vi "CH1_Comm_Stream.vi"   [LabVIEW 2018]
uses:
  RxTx/RxTx.lvclass
  Stream/Stream.lvclass
  Stream/Stream.lvclass/Stream.ctl
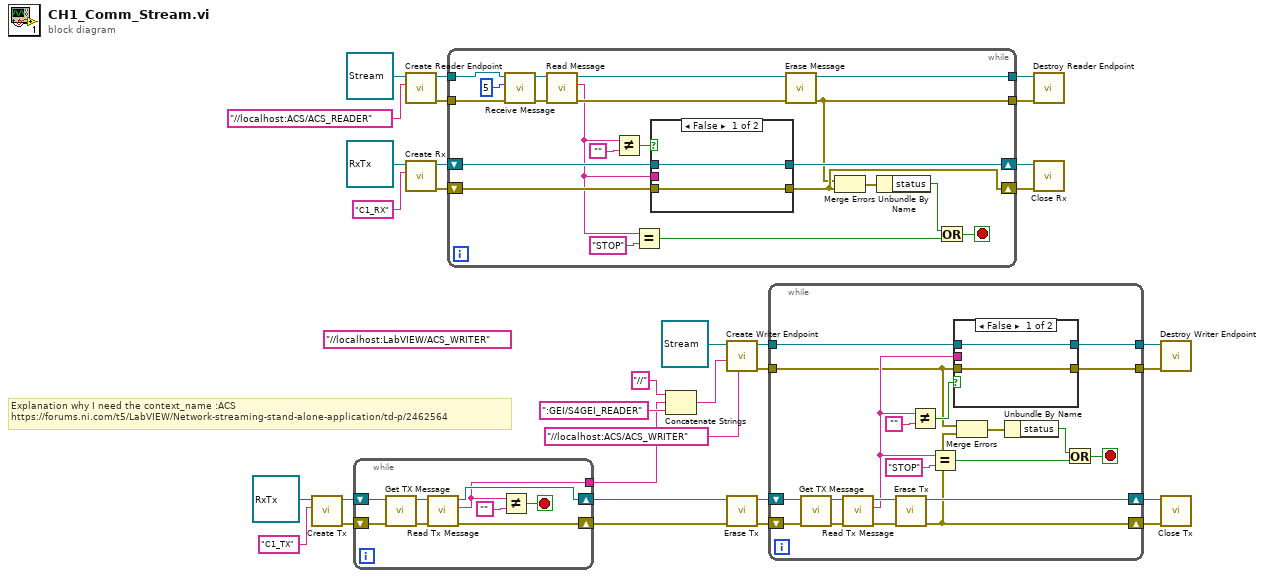
[diagram p0: block diagram]
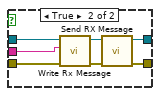
[diagram p2: hidden frame]
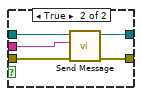
[diagram p3: hidden frame]
diagram:
  (unwired) "//localhost:LabVIEW/ACS_WRITER" ("reader name")
  # "Explanation why I need the context_name :ACS\nhttps://forums.ni.com/t5/LabVIEW/Network-streaming-stand-alone-application/td-p/2462564"
  n1 = call "Create Tx.vi"("Writer Name"="C1_TX", "RxTx in"=refnum<class "RxTx.lvclass"> refnum ("RxTx.lvclass")) -> ("error out"=w3:errorcluster, "RxTx out"=w2:refnum<class "RxTx.lvclass">)  [unwired: 8 in]
  n2 = while {
    shift-right: [w39] -> w4
    shift-left: w2 -> [w41]
    shift-right: [w38] -> w5
    shift-left: w3 -> [w36]
    tunnel: [w33] -> w1
    stop <- w34 stop-if-true
    n3 = call "Get TX Message.vi"("error in (no error)"=w36, "RxTx in"=w41) -> ("error out"=w37:errorcluster, "RxTx out"=w40:refnum<class "RxTx.lvclass">)  [unwired: 8 in]
    n4 = call "Read Tx Message.vi"("error in (no error)"=w37, "RxTx in"=w40) -> ("error out"=w38:errorcluster, "Tx Message"=w33:string, "RxTx out"=w39:refnum<class "RxTx.lvclass">)  [unwired: 7 in]
    n5 = Not Equal?(x=w33, y="") -> (x != y?=w34:bool)
  }
  n6 = call "Create Reader Endpoint.vi"("reader name"="//localhost:ACS/ACS_READER", "Stream in"=refnum<class "Stream.lvclass"> refnum) -> ("error out"=w25:errorcluster, "Stream out"=w26:refnum<class "Stream.lvclass">)  [unwired: 8 in]
  n7 = call "Create Rx.vi"("Reader Name"="C1_RX", "RxTx in"=refnum<class "RxTx.lvclass"> refnum ("RxTx.lvclass")) -> ("error out"=w11:errorcluster, "RxTx out"=w12:refnum<class "RxTx.lvclass">)  [unwired: 8 in]
  n8 = while {
    shift-right: [w60] -> w29
    shift-left: w12 -> [w62]
    shift-right: [w46] -> w30
    shift-left: w11 -> [w61]
    tunnel: w26 -> [w59]
    tunnel: w25 -> [w58]
    tunnel: [w52] -> w24
    tunnel: [w45] -> w23
    stop <- w42 stop-if-true
    n9 = call "Receive Message.vi"("error in (no error)"=w58, "timeout ms"=5, "Stream in"=w59) -> ("error out"=w55:errorcluster, "Stream out"=w56:refnum<class "Stream.lvclass">)  [unwired: 7 in]
    n10 = call "Read Message.vi"("error in (no error)"=w55, "Stream in"=w56) -> ("error out"=w53:errorcluster, "Message"=w48:string, "Stream out"=w54:refnum<class "Stream.lvclass">)  [unwired: 7 in]
    n11 = Not Equal?(x=w48, y="") -> (x != y?=w50:bool)
    n12 = Equal?(x=w48, y="STOP" ("reader name")) -> (x = y?=w47:bool)
    n13 = case shown="False" w50 {
      tunnel: w62 -> [w64 w71]
      tunnel: w61 -> [w63 w68]
      tunnel: [w63 w67] -> w46
      tunnel: [w64 w66] -> w60
      tunnel: w48 -> [_ w65]
      frame False {
      }
      frame True {
        n14 = call "Write Rx Message.vi"("error in (no error)"=w68, "Rx Message"=w65, "RxTx in"=w71) -> ("error out"=w69:errorcluster, "RxTx out"=w70:refnum<class "RxTx.lvclass">)  [unwired: 7 in]
        n15 = call "Send RX Message.vi"("error in (no error)"=w69, "RxTx in"=w70) -> ("error out"=w67:errorcluster, "RxTx out"=w66:refnum<class "RxTx.lvclass">)  [unwired: 8 in]
      }
    }
    n16 = call "Erase Message.vi"("error in (no error)"=w53, "Stream in"=w54) -> ("error out"=w45:errorcluster, "Stream out"=w52:refnum<class "Stream.lvclass">)  [unwired: 8 in]
    n17 = Merge Errors(w45, w46) -> (w44:errorcluster)
    n18 = Unbundle By Name(w44) -> ("status"=w43:bool)
    n19 = Or(x=w43, y=w47) -> (x .or. y?=w42:bool)
  }
  n20 = Concatenate Strings("//" ("reader name"), w1, ":GEI/S4GEI_READER" ("reader name")) -> (w9:string)
  n21 = call "Create Writer Endpoint.vi"("writer name"="//localhost:ACS/ACS_WRITER" ("reader name"), "reader name"=w9, "Stream in"=refnum<class "Stream.lvclass"> refnum) -> ("error out"=w21:errorcluster, "Stream out"=w22:refnum<class "Stream.lvclass">)  [unwired: 7 in]
  n22 = call "Erase Tx.vi"("error in (no error)"=w5, "RxTx in"=w4) -> ("error out"=w6:errorcluster, "RxTx out"=w7:refnum<class "RxTx.lvclass">)  [unwired: 8 in]
  n23 = while {
    shift-right: [w85] -> w31
    shift-left: w7 -> [w91]
    shift-right: [w74] -> w32
    shift-left: w6 -> [w90]
    tunnel: w22 -> [w82]
    tunnel: w21 -> [w73]
    tunnel: [w81] -> w20
    tunnel: [w80] -> w19
    stop <- w75 stop-if-true
    n24 = call "Get TX Message.vi"("error in (no error)"=w90, "RxTx in"=w91) -> ("error out"=w88:errorcluster, "RxTx out"=w89:refnum<class "RxTx.lvclass">)  [unwired: 8 in]
    n25 = call "Read Tx Message.vi"("error in (no error)"=w88, "RxTx in"=w89) -> ("error out"=w87:errorcluster, "Tx Message"=w79:string, "RxTx out"=w86:refnum<class "RxTx.lvclass">)  [unwired: 7 in]
    n26 = call "Erase Tx.vi"("error in (no error)"=w87, "RxTx in"=w86) -> ("error out"=w74:errorcluster, "RxTx out"=w85:refnum<class "RxTx.lvclass">)  [unwired: 8 in]
    n27 = Not Equal?(x=w79, y="") -> (x != y?=w83:bool)
    n28 = Equal?(x=w79, y="STOP") -> (x = y?=w77:bool)
    n29 = case shown="False" w83 {
      tunnel: w79 -> [_ w98]
      tunnel: w82 -> [w93 w97]
      tunnel: w73 -> [w92 w96]
      tunnel: [w92 w95] -> w81
      tunnel: [w93 w94] -> w80
      frame False {
      }
      frame True {
        n30 = call "Send Message.vi"("error in (no error)"=w96, "Message"=w98, "Stream in"=w97) -> ("error out"=w95:errorcluster, "Stream out"=w94:refnum<class "Stream.lvclass">)  [unwired: 7 in]
      }
    }
    n31 = Merge Errors(w73, w74) -> (w72:errorcluster)
    n32 = Unbundle By Name(w72) -> ("status"=w76:bool)
    n33 = Or(x=w76, y=w77) -> (x .or. y?=w75:bool)
  }
  n34 = call "Destroy Reader Endpoint.vi"("error in (no error)"=w23, "Stream in"=w24) -> ()  [unwired: 8 in, 2 out]
  n35 = call "Close Rx.vi"("error in (no error)"=w30, "RxTx in"=w29) -> ()  [unwired: 8 in, 2 out]
  n36 = call "Destroy Writer Endpoint.vi"("error in (no error)"=w20, "Stream in"=w19) -> ()  [unwired: 8 in, 2 out]
  n37 = call "Close Tx.vi"("error in (no error)"=w32, "RxTx in"=w31) -> ()  [unwired: 8 in, 2 out]
